vi "ImageData.vi"() -> (1 "Intensity vs Stage Position (mm)":cluster{dbl[], dbl[]}[](array[cluster]), 2 "Image intensities":dbl[](array[numeric]), 3 "Images":dbl[][][](array[numeric]))   [LabVIEW 2012]
uses:
  variables/GlobalUI.vi
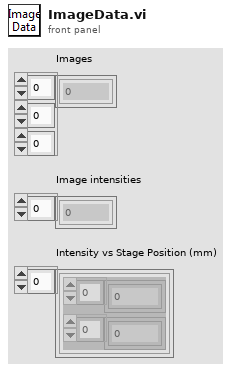
[diagram p1: front panel]
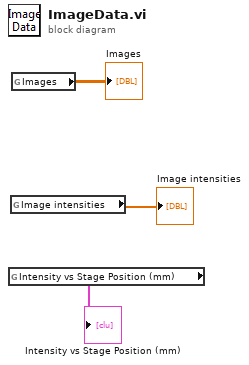
[diagram p0: block diagram]
diagram:
  n1 = global read "GlobalUI.vi" "Intensity vs Stage Position (mm)"() -> (→"Intensity vs Stage Position (mm)":cluster{dbl[], dbl[]}[])
  n2 = global read "GlobalUI.vi" "Image intensities"() -> (→"Image intensities":dbl[])
  n3 = global read "GlobalUI.vi" "Images"() -> (→"Images":dbl[][][])
